vi "json_raise_error.vi"(7 "message":string, 8 "error in (no error)":errorcluster, 11 "json":string) -> (0 "error out":errorcluster)   [LabVIEW 2017, in "rethinkdb.lvlib"]
uses:
  rethinkdb.lvlib
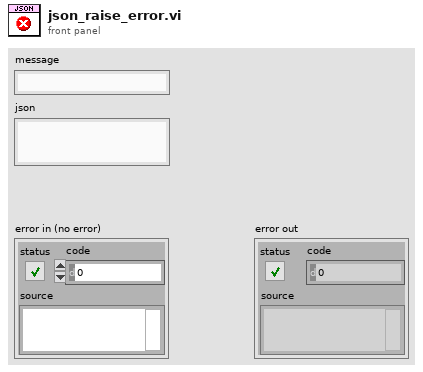
[diagram p1: front panel]
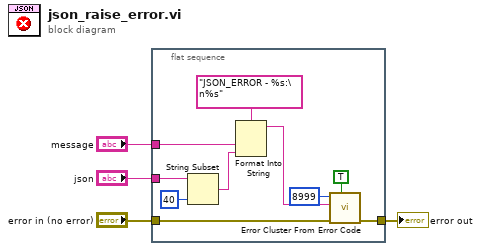
[diagram p0: block diagram]
diagram:
  n1 = flat-sequence {
    tunnel: "error in (no error)" -> [w14]
    tunnel: [w11] -> w3
    tunnel: "json" -> [w10]
    tunnel: "message" -> [w8]
    frame #0 {
      n2 = String Subset(string=w10, length (rest)=40 ("length (rest)")) -> (substring=w6:string)  [unwired: 1 in]
      n3 = Format Into String(format string="JSON_ERROR - %s:\n%s", w8, w6) -> (resulting string=w5:string)  [unwired: 2 in, 1 out]
      n4 = call <vilib>:"Error Cluster From Error Code.vi"("show call chain? (False)"=TRUE, "error in (no error)"=w14, "error message (\"\")"=w5, "error code (0)"=8999) -> ("error out"=w11:errorcluster)  [unwired: 5 in]
    }
  }
  "error out" <- w3
